vi "run_images.vi"(8 "error in (no error)":errorcluster, 11 "AnalysisRAPS in":refnum<class "AnalysisRAPS.lvclass">) -> (0 "error out":errorcluster, 3 "AnalysisRAPS out":refnum<class "AnalysisRAPS.lvclass">)   [LabVIEW 2010, in "AnalysisRAPS.lvclass"]
uses:
  AnalysisRAPS.lvclass
  common/classes/ErrorController/ErrorController/ErrorController.lvclass
  common/classes/Image/Image/Image.lvclass
  AnalysisRAPS.lvclass/AnalysisRAPS.ctl
  saving_type.ctl
  common/classes/ErrorController/ErrorController/class_data.vi
panel:
  out "error handler":bool
  in  "average":i32=1 min=1 step=1
  in  "button:stop":bool
  in  "Path":path
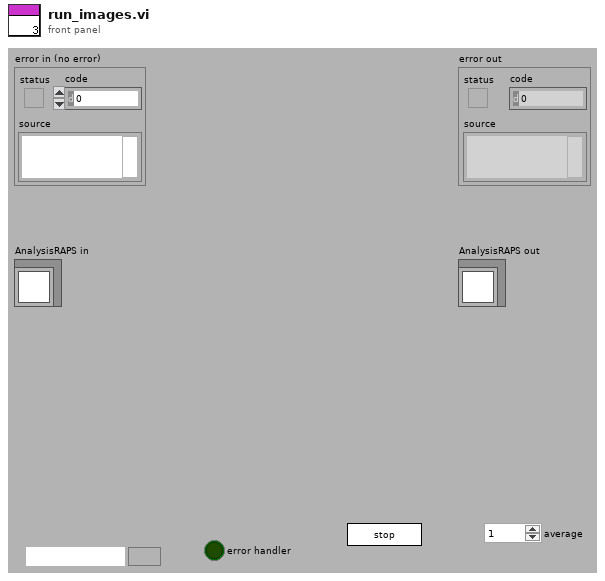
[diagram p1: front panel]
types:
  T1 = typedef "AnalysisRAPS.lvclass/saving_type.ctl" = enum16{"raw", "average"}
  T2 = typedef "Image Type" = u32
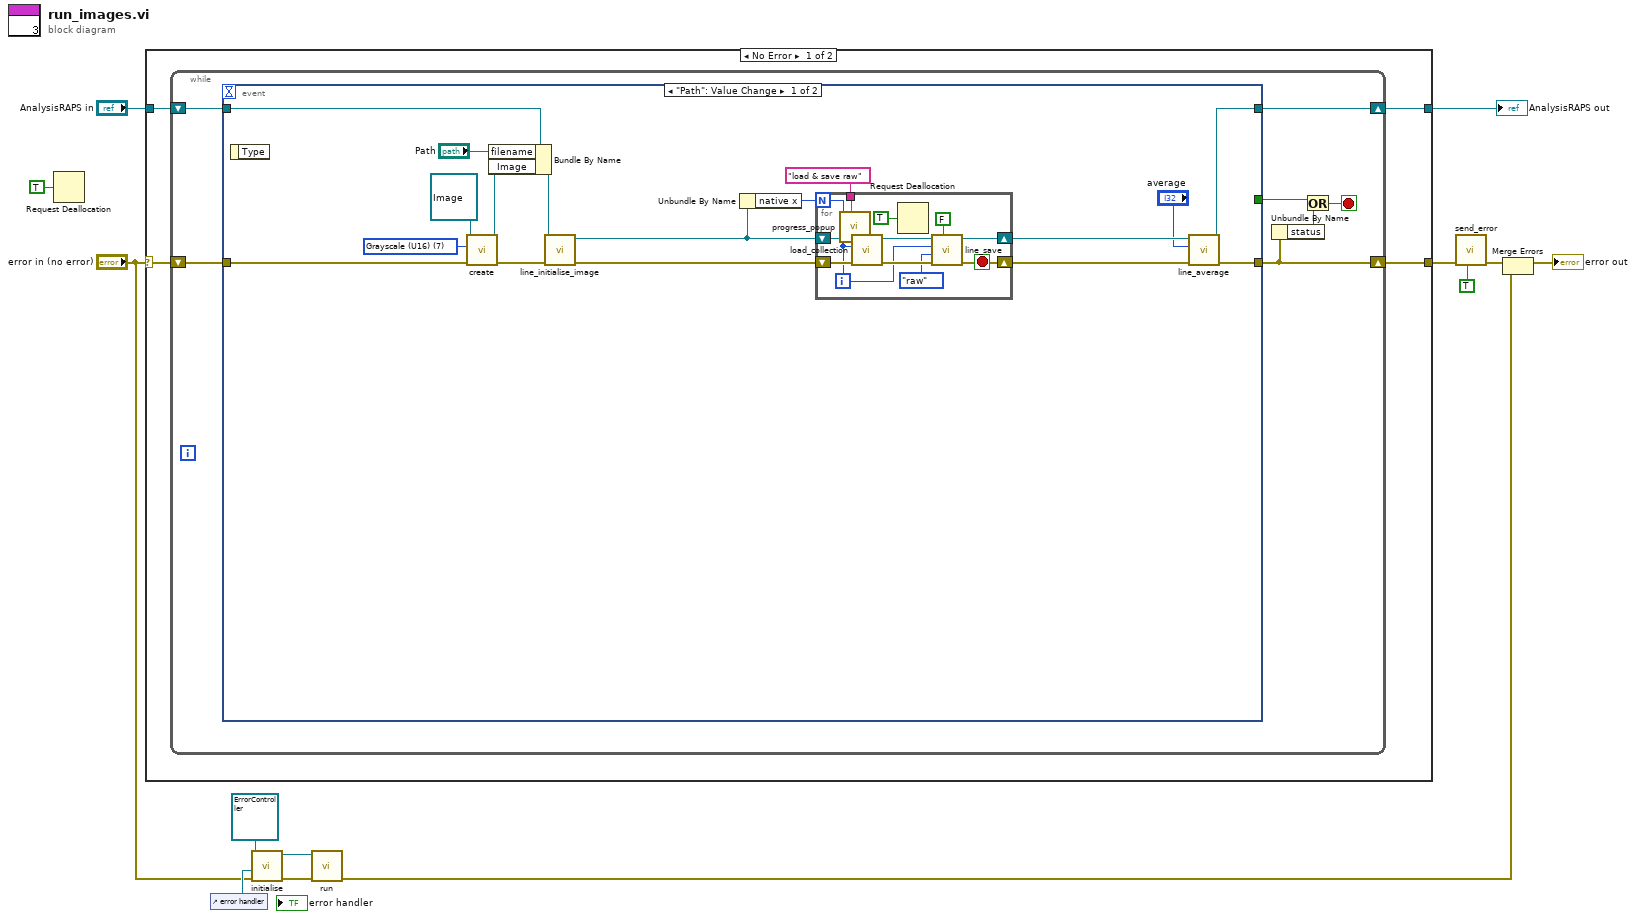
[diagram p0: block diagram]
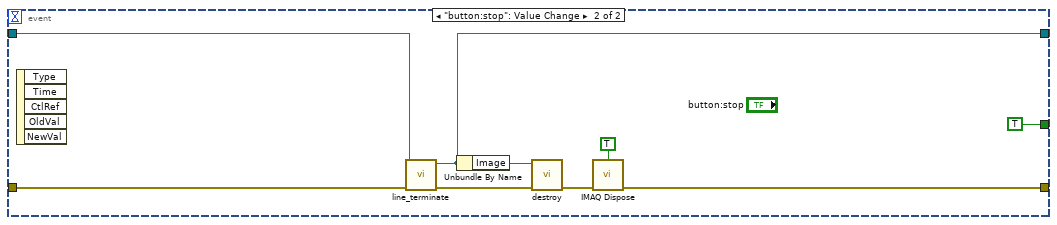
[diagram p2: hidden frame]
diagram:
  n1 = Request Deallocation(TRUE ("flag")) -> ()
  n2 = case shown="No Error" "error in (no error)" {
    selector: "error in (no error)" -> [w16 w64]
    tunnel: [w17 w64] -> w3
    tunnel: [w15 w63] -> w12
    tunnel: "AnalysisRAPS in" -> [w14 w63]
    frame No Error {
      n3 = while {
        shift-right: [w21] -> w17
        shift-left: w16 -> [w24]
        shift-right: [w23] -> w15
        shift-left: w14 -> [w22]
        stop <- w19 stop-if-true
        n4 = event shown="[0] \"Path\": Value Change" {
          selector: _ -> [_ _]
          dyn-events: _ -> [_ _]
          timeout: _ -> [_ _]
          tunnel: [w37 w58] -> w21
          tunnel: w24 -> [w32 w59]
          tunnel: [w39 w60] -> w23
          tunnel: w22 -> [w41 w61]
          tunnel: [_ TRUE] -> w18
          event "Path": Value Change {
            w33 = T2 7 items=["Grayscale (U8)", "Grayscale (I16)", "Grayscale (SGL)", "Complex (CSG)", "RGB (U32)", "HSL (U32)", "RGB (U64)", "Grayscale (U16)"] ("Image Type")
            n5 = event-data() -> ()  [unwired: 1 in, 1 out]
            n6 = call "create.vi"("error in (no error)"=w32, "Image Type"=w33, "Image in"=refnum<class "Image.lvclass"> refnum ("Image.lvclass")) -> ("error out"=w28:errorcluster, "Image out"=w30:refnum<class "Image.lvclass">)  [unwired: 7 in]
            n7 = Bundle By Name(cluster=w41, "filename"="Path", "Image"=w30) -> (w29:refnum<class "AnalysisRAPS.lvclass">)
            n8 = call-dynamic "line_initialise_image.vi"("error in (no error)"=w28, "AnalysisRAPS in"=w29) -> ("error out"=w27:errorcluster, "AnalysisRAPS out"=w26:refnum<class "AnalysisRAPS.lvclass">)  [unwired: 8 in]
            n9 = Unbundle By Name(w26) -> ("native x"=w25:i32)
            n10 = for {
              N: w25 -> [w47]
              shift-right: [w50] -> w40
              shift-left: w26 -> [w53]
              shift-right: [w48] -> w38
              shift-left: w27 -> [w52]
              tunnel: "load & save raw" -> [w45]
              i -> [w46]
              stop <- w48 stop-if-true
              n11 = call "progress_popup.vi"("custom text"=w45, "current"=w46, "total"=w47) -> ()  [unwired: 9 in]
              n12 = call-dynamic "load_collection.vi"("error in (no error)"=w52, "index"=w46, "AnalysisRAPS in"=w53) -> ("error out"=w49:errorcluster, "AnalysisRAPS out"=w51:refnum<class "AnalysisRAPS.lvclass">)  [unwired: 7 in]
              n13 = Request Deallocation(TRUE ("flag")) -> ()
              n14 = call-dynamic "line_save.vi"("double? (F)"=FALSE, "error in (no error)"=w49, "save type"=saving_type."raw", "index"=w46, "AnalysisRAPS in"=w51) -> ("error out"=w48:errorcluster, "AnalysisRAPS out"=w50:refnum<class "AnalysisRAPS.lvclass">)  [unwired: 5 in]
            }
            n15 = call-dynamic "line_average.vi"("error in (no error)"=w38, "average"="average", "AnalysisRAPS in"=w40) -> ("error out"=w37:errorcluster, "AnalysisRAPS out"=w39:refnum<class "AnalysisRAPS.lvclass">)  [unwired: 7 in]
          }
          event "button:stop": Value Change {
            n16 = event-data() -> ()  [unwired: 1 in, 5 out]
            n17 = call-dynamic "line_terminate.vi"("error in (no error)"=w59, "AnalysisRAPS in"=w61) -> ("error out"=w56:errorcluster, "AnalysisRAPS out"=w60:refnum<class "AnalysisRAPS.lvclass">)  [unwired: 8 in]
            n18 = Unbundle By Name(w60) -> ("Image"=w54:refnum<class "Image.lvclass">)
            n19 = call-dynamic "destroy.vi"("error in (no error)"=w56, "Image in"=w54) -> ("error out"=w55:errorcluster)  [unwired: 8 in, 1 out]
            n20 = call "IMAQ Dispose"("All Images? (No)"=TRUE, "error in (no error)"=w55) -> ("error out"=w58:errorcluster)  [unwired: 4 in]
          }
        }
        n21 = Unbundle By Name(w21) -> ("status"=w20:bool)
        n22 = Or(x=w18, y=w20) -> (x .or. y?=w19:bool)
      }
    }
    frame Error {
    }
  }
  "AnalysisRAPS out" <- w12
  n23 = control-ref of="error handler"() -> (w9:refnum<vi>)
  n24 = call-dynamic "initialise.vi"("error in (no error)"="error in (no error)", "error boolean"=w9, "ErrorController in"=refnum<class "ErrorController.lvclass"> refnum ("ErrorController.lvclass")) -> ("error out"=w7:errorcluster, "ErrorController out"=w6:refnum<class "ErrorController.lvclass">)  [unwired: 7 in]
  n25 = call "run.vi"("error in (no error)"=w7, "ErrorController in"=w6) -> ("error out"=w1:errorcluster)  [unwired: 8 in, 1 out]
  n26 = call "send_error.vi"("last error? (F)"=TRUE, "error in (no error)"=w3) -> ("error out"=w5:errorcluster)  [unwired: 9 in]
  n27 = Merge Errors(w5, w1) -> (→"error out":errorcluster)
